vi "Get Columns.vi"(8 "error in (no error)":errorcluster, 10 "Table Name":string, 11 "MS Access in":refnum<class "MS Access.lvclass">) -> (0 "error out":errorcluster, 2 "Column Name Array":string[](array[string]), 3 "MS Access out":refnum<class "MS Access.lvclass">)   [LabVIEW 2020, in "MS Access.lvclass"]
uses:
  MS Access.lvclass
  ODBC/ADODB.lvclass
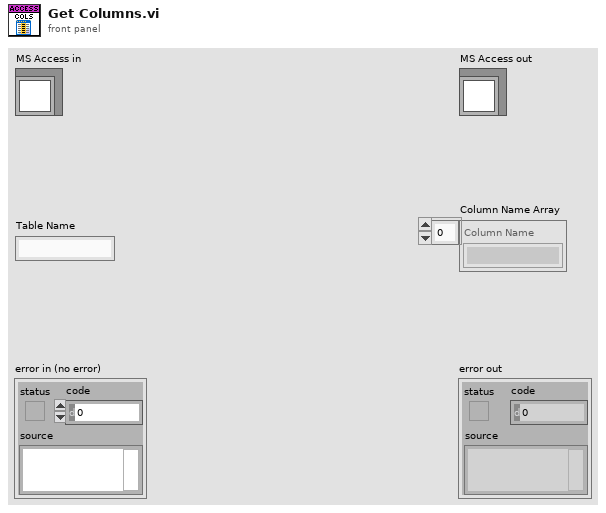
[diagram p1: front panel]
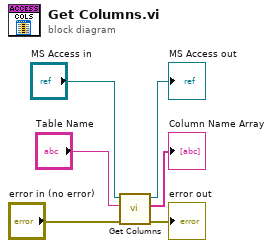
[diagram p0: block diagram]
diagram:
  n1 = call-parent "Get Columns.vi"("error in (no error)"="error in (no error)", "Table Name"="Table Name", "ODBC in"="MS Access in") -> ("error out"=→"error out":errorcluster, "Column Name Array"=→"Column Name Array":string[], "ODBC out"=→"MS Access out":refnum<class "MS Access.lvclass">)  [unwired: 6 in]
